vi "HysteresisControl.vi"(0 "Process variable":dbl, 1 "Low threshold":dbl, 2 "High threshold":dbl, 3 "Run in":bool, 4 "Start":bool) -> (5 "Run out":bool)   [LabVIEW 2020]
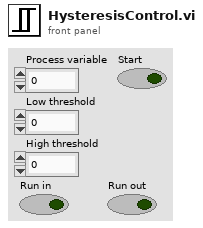
[diagram p1: front panel]
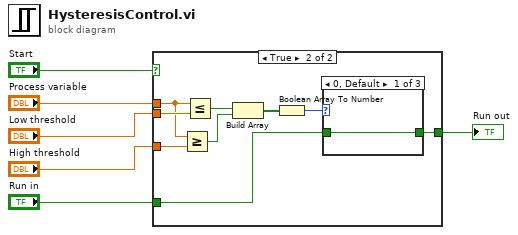
[diagram p0: block diagram]
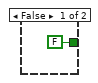
[diagram p2: hidden frame]
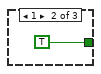
[diagram p3: hidden frame]
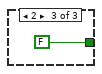
[diagram p4: hidden frame]
diagram:
  n1 = case shown="True" "Start" {
    tunnel: "Low threshold" -> [_ w16]
    tunnel: "High threshold" -> [_ w15]
    tunnel: "Process variable" -> [_ w8]
    tunnel: [FALSE ("Run in") w10] -> w5
    tunnel: "Run in" -> [_ w9]
    frame False {
    }
    frame True {
      n2 = Greater Or Equal?(x=w8, y=w15) -> (x >= y?=w13:bool)
      n3 = Less Or Equal?(x=w8, y=w16) -> (x <= y?=w14:bool)
      n4 = Build Array(w14, w13) -> (w12:bool[])
      n5 = Boolean Array To Number(Boolean array=w12) -> (number=w11:u32)
      n6 = case shown="0, Default" w11 {
        tunnel: [w17 TRUE FALSE] -> w10
        tunnel: w9 -> [w17 _ _]
        frame 0, Default {
        }
        frame 1 {
        }
        frame 2 {
        }
      }
    }
  }
  "Run out" <- w5
